vi "AutonomousDataWire.vi"(10 "String in":string, 11 "Number in":string) -> (2 "Number out":string, 3 "String out":string="N/A")   [LabVIEW 2015]
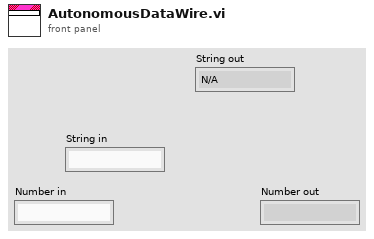
[diagram p1: front panel]
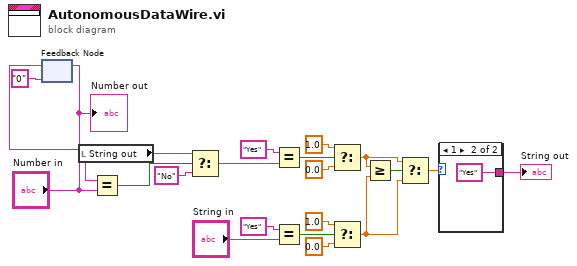
[diagram p0: block diagram]
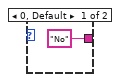
[diagram p2: hidden frame]
diagram:
  n1 = feedback #1("0" ("Number in")) -> (w5:string)
  n2 = feedback-in #1("Number in") -> ()
  n3 = local read "String out"() -> (w1:string)
  n4 = Equal?(x=w5, y="Number in") -> (x = y?=w3:bool)
  n5 = Select(t=w1, s=w3, f="No" ("x")) -> (s? t:f=w9:string)
  n6 = Equal?(x="Yes", y=w9) -> (x = y?=w17:bool)
  n7 = Equal?(x="Yes", y="String in") -> (x = y?=w11:bool)
  n8 = Select(t=1.0, s=w17, f=0.0) -> (s? t:f=w8:dbl)
  n9 = Select(t=1.0, s=w11, f=0.0) -> (s? t:f=w7:dbl)
  n10 = Greater Or Equal?(x=w8, y=w7) -> (x >= y?=w19:bool)
  n11 = Select(t=w8, s=w19, f=w7) -> (s? t:f=w20:dbl)
  n12 = case shown="1" w20 {
    tunnel: ["No" ("x") "Yes" ("x")] -> w21
    frame 0, Default {
    }
    frame 1 {
    }
  }
  "String out" <- w21
  "Number out" <- "Number in"
